vi "salRegSubEventsDtApp.vi"(8 "error in (no error)":errorcluster, 11 "MiddlewareSALThisComponent in":refnum<class "MiddlewareSALThisComponent.lvclass">) -> (0 "error out":errorcluster, 2 "SAL Event Reg Refnum":refnum<event-registration>, 3 "MiddlewareSALThisComponent out":refnum<class "MiddlewareSALThisComponent.lvclass">)   [LabVIEW 2016, in "MiddlewareSALThisComponent.lvclass"]
uses:
  MiddlewareSALThisComponent.lvclass
  <vilib>/Utility/error.llb/DialogType.ctl
  ts_sallv_exa/SALLV_EXA.lvlib
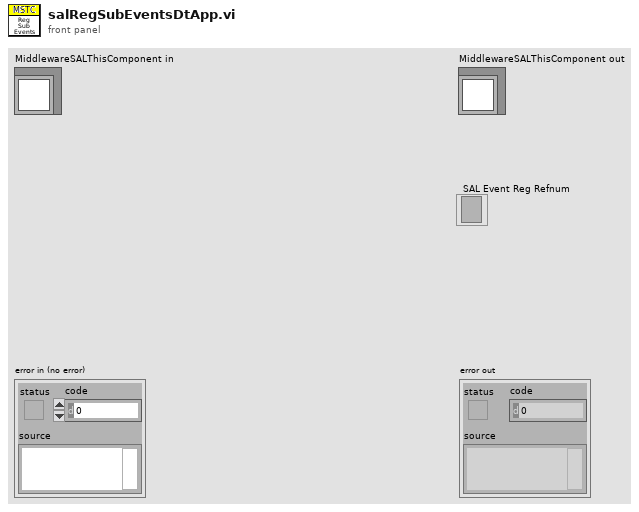
[diagram p1: front panel]
types:
  T1 = typedef "DialogType.ctl" = u16
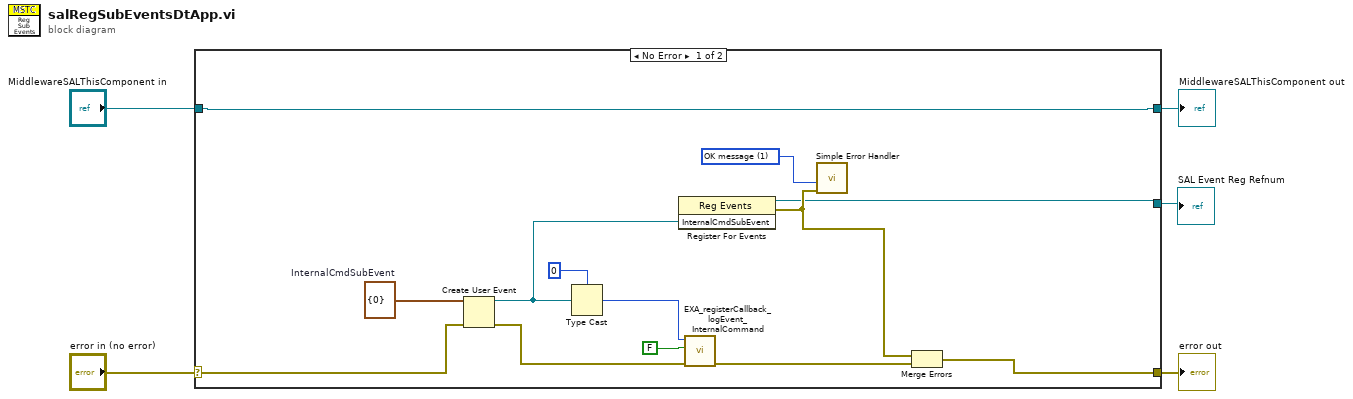
[diagram p0: block diagram]
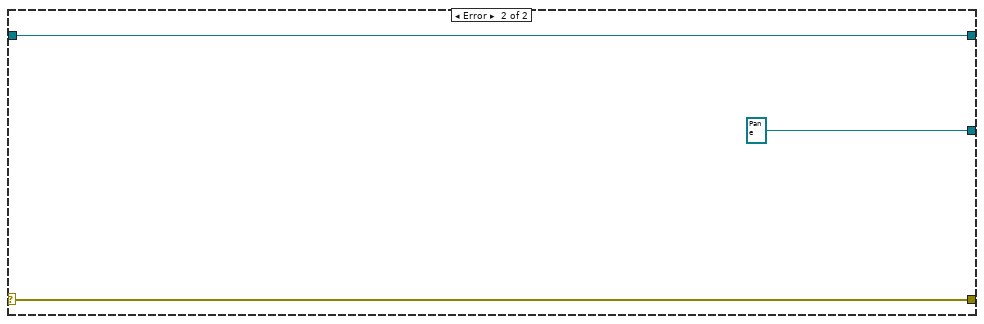
[diagram p2: hidden frame]
diagram:
  n1 = case shown="No Error" "error in (no error)" {
    selector: "error in (no error)" -> [w6 w21]
    tunnel: [w8 w21] -> w4
    tunnel: [w18 w20] -> w2
    tunnel: "MiddlewareSALThisComponent in" -> [w18 w20]
    tunnel: [w7 refnum<event-registration> refnum ("Event Registration Refnum")] -> w1
    frame No Error {
      w11 = cluster{"Data":i32} {"Data"=0}  # InternalCmdSubEvent
      w17 = T1 1 items=["no dialog", "OK message", "continue or stop message", "OK message + warnings", "continue/stop + warnings"] ("type of dialog (OK msg:1)")
      n2 = Create User Event(user event datatype=w11, error in=w6) -> (user event=w10:refnum<user-event>, error out=w9:errorcluster)
      n3 = Type Cast(type=0, x=w10) -> (*(type *) &x=w14:i32)
      n4 = register-events(w10) -> (reference out=w7:refnum<event-registration>, error out=w13:errorcluster)  [unwired: 2 in]
      n5 = call "EXA_registerCallback_logEvent_InternalCommand.vi"("error in (no error)"=w9, "skipOld"=FALSE, "handle"=w14) -> ("error out"=w12:errorcluster)  [unwired: 7 in, 1 out]
      n6 = call <vilib>:"Simple Error Handler.vi"("type of dialog (OK msg:1)"=w17, "error in (no error)"=w13) -> ()  [unwired: 3 in, 5 out]
      n7 = Merge Errors(w13, w12) -> (w8:errorcluster)
    }
    frame Error {
    }
  }
  "error out" <- w4
  "MiddlewareSALThisComponent out" <- w2
  "SAL Event Reg Refnum" <- w1
